vi "Free Running Avs47b With Autoranging.vi"() -> ()   [LabVIEW 2012]
doc: "Application example"
panel:
  in  "REMOTE":enum16{"DISABLED", "ENABLED"}(ring)
  out "UNDERRANGE":bool
  in  "AUTORANGE":enum16{"DISABLED", "ENABLED"}(ring)
  in  "stop":bool
  out "RESISTANCE":sgl format="%^_6e"
  in  "EXCITATION":u8(ring)=7 items=["NO EXCITATION", "3 uV", "10uV", "30uV", "100uV", "300uV", "1mV", "3mV"]
  in  "RANGE":u8(ring)=1 items=["NO RANGE", "2 Ohms", "20 Ohms", "200 Ohms", "2 kOhms", "20 kOhms", "200 kOhms", "2 MOhms"]
  in  "CHANNEL":u8(ring) items=["CH0", "CH1", "CH2", "CH3", "CH4", "CH5", "CH6", "CH7"]
  in  "INPUT":u8(ring)=1 items=["ZERO", "MEAS", "CAL"]
  out "OVERRANGE":bool
  # "Free Running Avs47b With Autoranging.vi"
  # "Ohms"
  # "The VI starts using the following modes. Please\nselect them before starting to run the VI."
  # "This example adds autoranging to the free-running AVS-47B.  The autoranging.vi suggests a new\nlower or higher range if the ADC reading is below 1800 or over 19000.  Range is then changed,\nprovided, that the bridge is in remote mode and provided that there is a lower or higher range \navailable.\n\nPlease use autoranging works only in remote mode.  If used in local mode, range can make an\nunwanted jump, if remote is enabled later.\n\nUnlike in many other examples, this VI  has both overrange and underrange indicators. Both\nwork similarly regardless of whether autoranging is enabled or disabled. Underrange indicator is \nset if reading falls below 1800 and overrange indicator is set if reading exceeds 19000. These\nlimits provide some hysteresis and they are set in Autoranging.vi. \n\nIf the voltage to the A/D converter exceeds 1.9999 Volts, overrange indicator is set true while the \nADC reading is exact zero.  Therefore, all applications shall use overload indication either from\nthe Autoranging.vi or from the ADC so that the overload-zero reading can be separated from a \ntrue measured (almost) zero resistance."
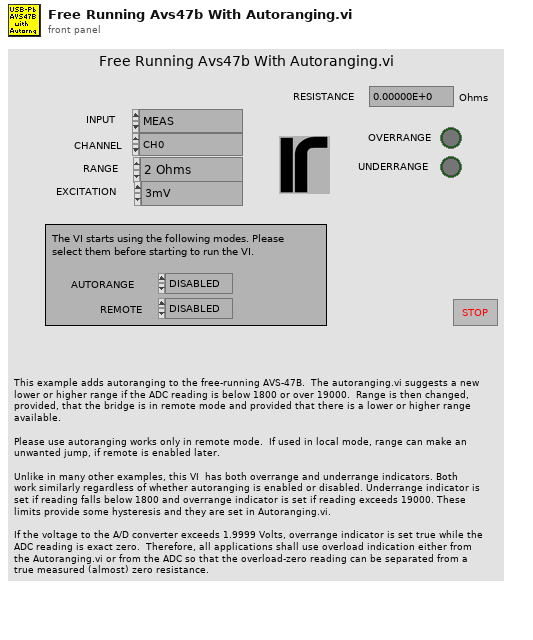
[diagram p1: front panel]
types:
  T1 = cluster{"VISA RESOURCE":refnum<visa-resource-name>, "PICOBUS ADDRESS":u8, "DISABLE AL":u8, "REMOTE":u8, "INPUT":u8, "CHANNEL":u8, "RANGE":u8, "EXCITATION":u8, "DISPLAY":u8, "DIGITAL REFERENCE":u16, "SET POINT":dbl, "PROP GAIN":u8, "INTG":u8, "DERIV":u8, "POWER BIAS":u8, "POWER RANGE":u8, "INFO STRING":string, "HEATER RESISTANCE":dbl, "INTERVAL":u8, " SENSOR dR/dT":u8}
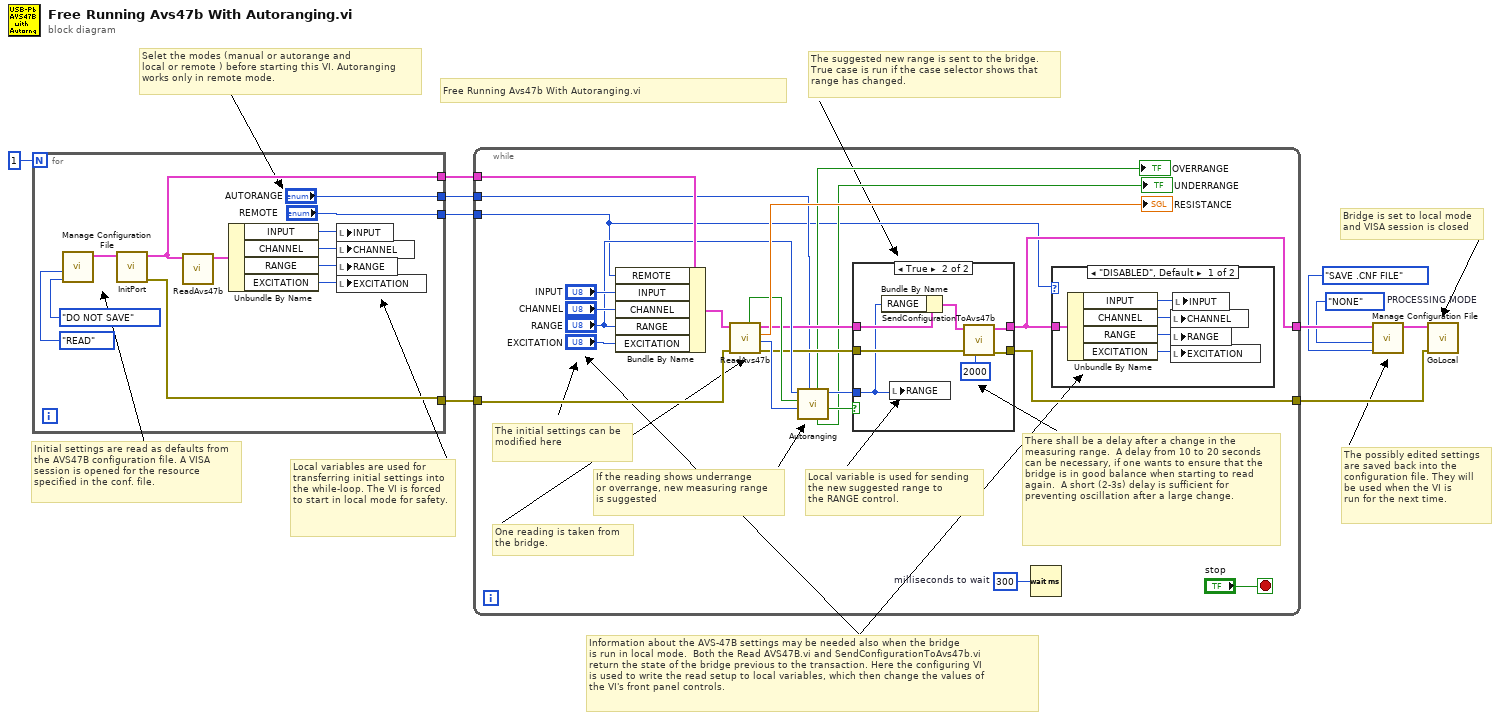
[diagram p0: block diagram]
diagram:
  w3 = enum16{"NONE", "READ", "CREATE"}."NONE"  # PROCESSING MODE
  # "Information about the AVS-47B settings may be needed also when the bridge\nis run in local mode.  Both the Read AVS47B.vi and SendConfigurationToAvs47b.vi\nreturn the state of the bridge previous to the transaction. Here the configuring VI\nis used to write the read setup to local variables, which then change the values of\nthe VI's front panel controls."
  # "Selet the modes (manual or autorange and \nlocal or remote ) before starting this VI. Autoranging \nworks only in remote mode."
  # "Bridge is set to local mode\nand VISA session is closed"
  # "The possibly edited settings\nare saved back into the \nconfiguration file. They will\nbe used when the VI is\nrun for the next time."
  # "Local variables are used for \ntransferring initial settings into\nthe while-loop. The VI is forced to start in local mode for safety."
  # "The suggested new range is sent to the bridge. \nTrue case is run if the case selector shows that\nrange has changed."
  # "Initial settings are read as defaults from\nthe AVS47B configuration file. A VISA\nsession is opened for the resource\nspecified in the conf. file."
  # "Free Running Avs47b With Autoranging.vi"
  n1 = for {
    N: 1 -> [_]
    tunnel: [w13] -> w9
    tunnel: [w12] -> w8
    tunnel: ["AUTORANGE"] -> w7
    tunnel: ["REMOTE"] -> w1
    n2 = call "Manage Configuration File.vi"("SAVE MODE"=enum16{"DO NOT SAVE", "SAVE .CNF FILE"}."DO NOT SAVE", "PROCESSING MODE"=enum16{"NONE", "READ", "CREATE"}."READ") -> ("CONFIGURATION CLUSTER OUT"=w14:T1)  [unwired: 9 in]
    n3 = call "InitPort.vi"("CONFIGURATION CLUSTER"=w14) -> ("LV ERROR OUT"=w13:errorcluster, "UNMODIFIED CONFIGURATION CLUSTER"=w12:T1)  [unwired: 6 in, 1 out]
    n4 = call "ReadAvs47b.vi"("CONFIGURATION CLUSTER"=w12) -> ("MODIFIED CONFIGURATION CLUSTER"=w22:T1)  [unwired: 5 in, 5 out]
    n5 = Unbundle By Name(w22) -> ("INPUT"=w21:u8, "CHANNEL"=w20:u8, "RANGE"=w19:u8, "EXCITATION"=w18:u8)
    n6 = local write "INPUT"(w21) -> ()
    n7 = local write "CHANNEL"(w20) -> ()
    n8 = local write "RANGE"(w19) -> ()
    n9 = local write "EXCITATION"(w18) -> ()
  }
  n10 = while {
    tunnel: w9 -> [w44]
    tunnel: [w26] -> w5
    tunnel: w8 -> [w38]
    tunnel: w7 -> [w25]
    tunnel: [w24] -> w4
    tunnel: w1 -> [w23]
    stop <- "stop" stop-if-true
    w43 = u32 300  # milliseconds to wait
    # "There shall be a delay after a change in the measuring range.  A delay from 10 to 20 seconds can be necessary, if one wants to ensure that the bridge is in good balance when starting to read again.  A short (2-3s) delay is sufficient for preventing oscillation after a large change."
    # "Local variable is used for sending\nthe new suggested range to\nthe RANGE control."
    # "If the reading shows underrange\nor overrange, new measuring range\nis suggested"
    # "One reading is taken from\nthe bridge."
    # "The initial settings can be modified here"
    n11 = Bundle By Name(cluster=w38, "REMOTE"=w23, "INPUT"="INPUT", "CHANNEL"="CHANNEL", "RANGE"="RANGE", "EXCITATION"="EXCITATION") -> (w42:T1)
    n12 = call "ReadAvs47b.vi"("LV ERROR IN"=w44, "CONFIGURATION CLUSTER"=w42) -> ("LV ERROR OUT"=w32:errorcluster, "ADC"=w34:i32, "RESISTANCE (OHMS)"=→"RESISTANCE":sgl, "MODIFIED CONFIGURATION CLUSTER"=w29:T1, "ADC OVERRANGE"=w35:bool)  [unwired: 4 in, 1 out]
    n13 = call "Autoranging.vi"("AUTORANGE"=w25, "ADC"=w34, "OVR"=w35, "RANGE"="RANGE") -> ("RANGE HAS CHANGED"=w31:bool, "NEW RANGE"=w30:i32, "UNDERRANGE"=→"UNDERRANGE":bool, "OVERRANGE"=→"OVERRANGE":bool)  [unwired: 4 in]
    n14 = case shown="True" w31 {
      tunnel: [w51 w57] -> w26
      tunnel: w32 -> [w50 w55]
      tunnel: [w50 w54] -> w24
      tunnel: w30 -> [_ w52]
      tunnel: w29 -> [w51 w58]
      frame False {
      }
      frame True {
        n15 = Bundle By Name(cluster=w58, "RANGE"=w52) -> (w56:T1)
        n16 = local write "RANGE"(w52) -> ()
        n17 = call "SendConfigurationToAvs47b.vi"("STABILISATION DELAY (ms)"=2000, "LV ERROR IN"=w55, "CONFIGURATION CLUSTER"=w56) -> ("LV ERROR OUT"=w54:errorcluster, "UNMODIFIED CONFIGURATION CLUSTER"=w57:T1)  [unwired: 5 in, 2 out]
      }
    }
    n18 = Wait (ms)(milliseconds to wait=w43) -> ()  [unwired: 1 out]
    n19 = case shown="\"DISABLED\", Default" w23 {
      tunnel: w26 -> [w49 _]
      frame "DISABLED", Default {
        n20 = Unbundle By Name(w49) -> ("INPUT"=w48:u8, "CHANNEL"=w47:u8, "RANGE"=w46:u8, "EXCITATION"=w45:u8)
        n21 = local write "CHANNEL"(w47) -> ()
        n22 = local write "RANGE"(w46) -> ()
        n23 = local write "EXCITATION"(w45) -> ()
        n24 = local write "INPUT"(w48) -> ()
      }
      frame "ENABLED" {
      }
    }
  }
  n25 = call "Manage Configuration File.vi"("SAVE MODE"=enum16{"DO NOT SAVE", "SAVE .CNF FILE"}."SAVE .CNF FILE", "PROCESSING MODE"=w3, "CONFIGURATION CLUSTER"=w5) -> ("CONFIGURATION CLUSTER OUT"=w6:T1)  [unwired: 8 in]
  n26 = call "GoLocal.vi"("LV ERROR IN"=w4, "CONFIGURATION CLUSTER"=w6) -> ()  [unwired: 9 in, 1 out]
